vi "single_pulse_config.vi"(1 "output cluster":T1) -> (0 "Error output":T2)   [LabVIEW 2015]
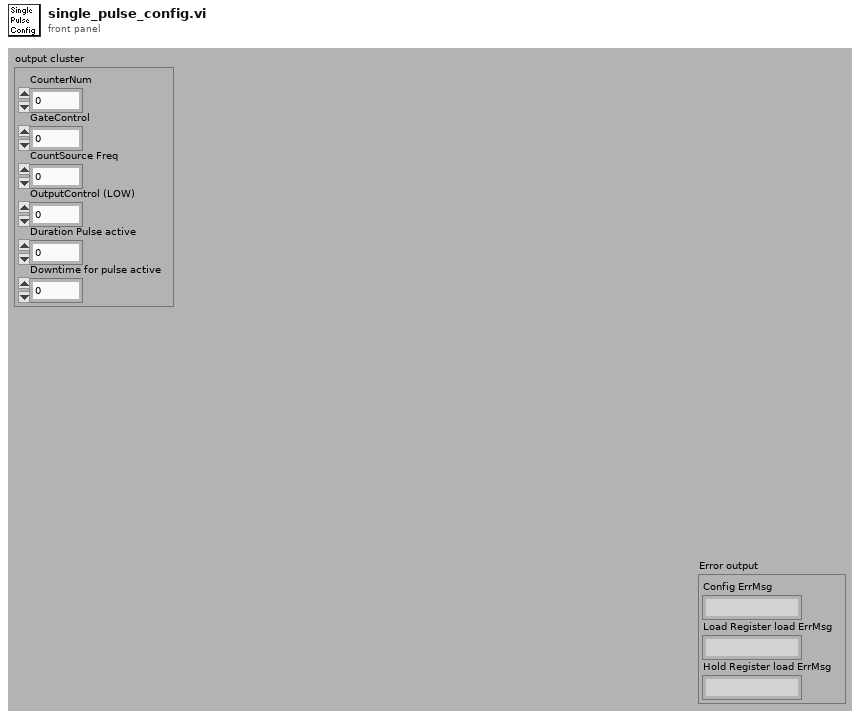
[diagram p1: front panel]
types:
  T1 = cluster{"CounterNum":u32, "GateControl":u32, "CountSource Freq":u32, "OutputControl (LOW)":u32, "Duration Pulse active":u32, "Downtime for pulse active":u32}
  T2 = cluster{"Config ErrMsg":string, "Load Register load ErrMsg":string, "Hold Register load ErrMsg":string}
  T3 = cluster{"ErrMsg":string, "ErrMsg":string, "ErrMsg":string}
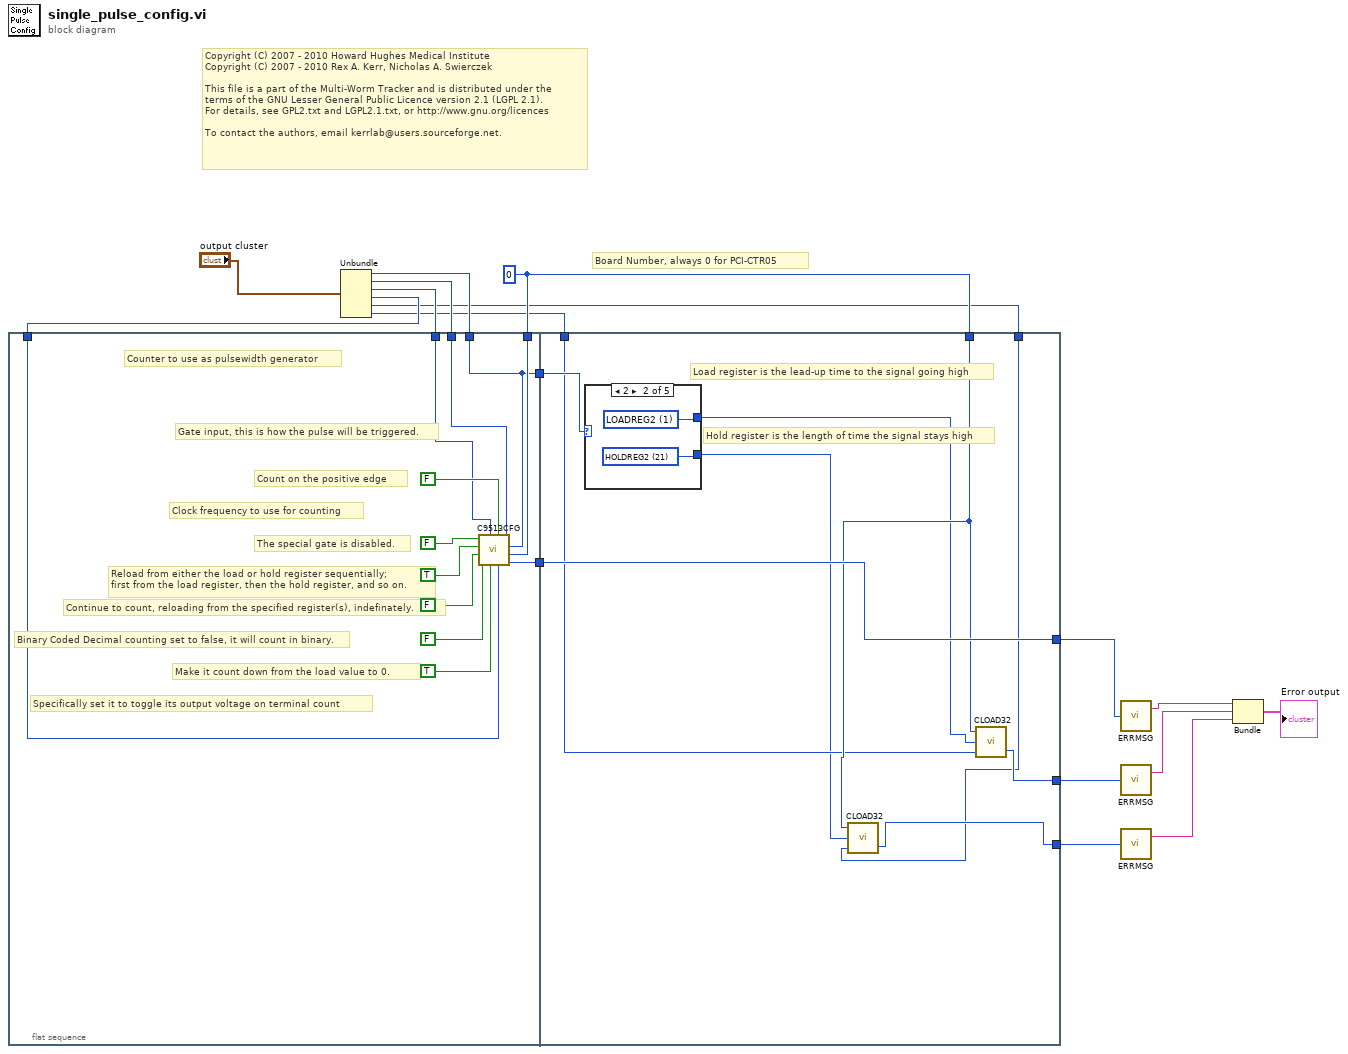
[diagram p0: block diagram]
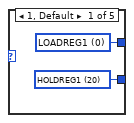
[diagram p2: hidden frame]
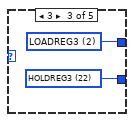
[diagram p3: hidden frame]
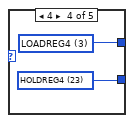
[diagram p4: hidden frame]
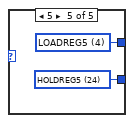
[diagram p5: hidden frame]
diagram:
  w9 = u32 0 ("BoardNum (0)")
  # "Copyright (C) 2007 - 2010 Howard Hughes Medical Institute\nCopyright (C) 2007 - 2010 Rex A. Kerr, Nicholas A. Swierczek\n \nThis file is a part of the Multi-Worm Tracker and is distributed under the\nterms of the GNU Lesser General Public Licence version 2.1 (LGPL 2.1).\nFor details, see GPL2.txt and LGPL2.1.txt, or http://www.gnu.org/licences\n \nTo contact the authors, email kerrlab@users.sourceforge.net."
  # "Board Number, always 0 for PCI-CTR05"
  n1 = flat-sequence {
    tunnel: [w23] -> w10
    tunnel: w9 -> [w22]
    tunnel: [w21] -> w8
    tunnel: w7 -> [w21]
    tunnel: w6 -> [w20]
    tunnel: w5 -> [w19]
    tunnel: w4 -> [w18]
    tunnel: [w38] -> w13
    tunnel: [w37] -> w12
    tunnel: [w36] -> w11
    tunnel: w10 -> [w36]
    tunnel: w9 -> [w35]
    tunnel: w8 -> [w33]
    tunnel: w3 -> [w32]
    tunnel: w2 -> [w31]
    frame #0 {
      # "Continue to count, reloading from the specified register(s), indefinately."
      # "Specifically set it to toggle its output voltage on terminal count"
      # "Make it count down from the load value to 0."
      # "Binary Coded Decimal counting set to false, it will count in binary."
      # "Reload from either the load or hold register sequentially;\nfirst from the load register, then the hold register, and so on."
      # "The special gate is disabled."
      # "Clock frequency to use for counting"
      # "Count on the positive edge"
      # "Gate input, this is how the pulse will be triggered."
      # "Counter to use as pulsewidth generator"
      n2 = call <menus>:"C9513CFG.VI"("BCDMode (DISABLED)"=FALSE, "CountDirection (UP)"=TRUE, "OutputControl (LOW)"=w18, "Recycle (ONETIME)"=FALSE, "BoardNum (0)"=w22, "Reload (LOADREG)"=TRUE, "CounterNum (1)"=w21, "SpecialGate (DISABLED)"=FALSE, "CountSource"=w19, "CountEdge(POSITIVE)"=FALSE, "GateControl"=w20) -> ("ErrCode"=w23:i32)
    }
    frame #1 {
      # "Load register is the lead-up time to the signal going high"
      # "Hold register is the length of time the signal stays high"
      n3 = case shown="2" w33 {
        tunnel: [w40 w42 w44 w46 w48] -> w34
        tunnel: [w39 w41 w43 w45 w47] -> w30
        frame 1, Default {
          w39 = u32 20 items=["LOADREG1", "LOADREG2", "LOADREG3", "LOADREG4", "LOADREG5", "LOADREG6", "LOADREG7", "LOADREG8", "LOADREG9", "LOADREG10", "LOADREG11", "LOADREG12", "LOADREG13", "LOADREG14", "LOADREG15", "LOADREG16", "LOADREG17", "LOADREG18", "LOADREG19", "LOADREG20", "HOLDREG1", "HOLDREG2", "HOLDREG3", "HOLDREG4", "HOLDREG5", "HOLDREG6", "HOLDREG7", "HOLDREG8", "HOLDREG9", "HOLDREG10", "HOLDREG11", "HOLDREG12", "HOLDREG13", "HOLDREG14", "HOLDREG15", "HOLDREG16", "HOLDREG17", "HOLDREG18", "HOLDREG19", "HOLDREG20", "ALARM1CHIP1", "ALARM2CHIP1", "ALARM1CHIP2", "ALARM2CHIP2", "ALARM1CHIP3", "ALARM2CHIP3", "ALARM1CHIP4", "ALARM2CHIP4", "COUNT1", "COUNT2", "COUNT3", "COUNT4", "PRESET1", "PRESET2", "PRESET3", "PRESET4", "PRESCALER1", "PRESCALER2", "PRESCALER3", "PRESCALER4"] ("Counter 1 Hold RegName")
          w40 = u32 0 items=["LOADREG1", "LOADREG2", "LOADREG3", "LOADREG4", "LOADREG5", "LOADREG6", "LOADREG7", "LOADREG8", "LOADREG9", "LOADREG10", "LOADREG11", "LOADREG12", "LOADREG13", "LOADREG14", "LOADREG15", "LOADREG16", "LOADREG17", "LOADREG18", "LOADREG19", "LOADREG20", "HOLDREG1", "HOLDREG2", "HOLDREG3", "HOLDREG4", "HOLDREG5", "HOLDREG6", "HOLDREG7", "HOLDREG8", "HOLDREG9", "HOLDREG10", "HOLDREG11", "HOLDREG12", "HOLDREG13", "HOLDREG14", "HOLDREG15", "HOLDREG16", "HOLDREG17", "HOLDREG18", "HOLDREG19", "HOLDREG20", "ALARM1CHIP1", "ALARM2CHIP1", "ALARM1CHIP2", "ALARM2CHIP2", "ALARM1CHIP3", "ALARM2CHIP3", "ALARM1CHIP4", "ALARM2CHIP4", "COUNT1", "COUNT2", "COUNT3", "COUNT4", "PRESET1", "PRESET2", "PRESET3", "PRESET4", "PRESCALER1", "PRESCALER2", "PRESCALER3", "PRESCALER4"] ("Counter 1 Load RegName")
        }
        frame 2 {
          w41 = u32 21 items=["LOADREG1", "LOADREG2", "LOADREG3", "LOADREG4", "LOADREG5", "LOADREG6", "LOADREG7", "LOADREG8", "LOADREG9", "LOADREG10", "LOADREG11", "LOADREG12", "LOADREG13", "LOADREG14", "LOADREG15", "LOADREG16", "LOADREG17", "LOADREG18", "LOADREG19", "LOADREG20", "HOLDREG1", "HOLDREG2", "HOLDREG3", "HOLDREG4", "HOLDREG5", "HOLDREG6", "HOLDREG7", "HOLDREG8", "HOLDREG9", "HOLDREG10", "HOLDREG11", "HOLDREG12", "HOLDREG13", "HOLDREG14", "HOLDREG15", "HOLDREG16", "HOLDREG17", "HOLDREG18", "HOLDREG19", "HOLDREG20", "ALARM1CHIP1", "ALARM2CHIP1", "ALARM1CHIP2", "ALARM2CHIP2", "ALARM1CHIP3", "ALARM2CHIP3", "ALARM1CHIP4", "ALARM2CHIP4", "COUNT1", "COUNT2", "COUNT3", "COUNT4", "PRESET1", "PRESET2", "PRESET3", "PRESET4", "PRESCALER1", "PRESCALER2", "PRESCALER3", "PRESCALER4"] ("Counter 1 Hold RegName")
          w42 = u32 1 items=["LOADREG1", "LOADREG2", "LOADREG3", "LOADREG4", "LOADREG5", "LOADREG6", "LOADREG7", "LOADREG8", "LOADREG9", "LOADREG10", "LOADREG11", "LOADREG12", "LOADREG13", "LOADREG14", "LOADREG15", "LOADREG16", "LOADREG17", "LOADREG18", "LOADREG19", "LOADREG20", "HOLDREG1", "HOLDREG2", "HOLDREG3", "HOLDREG4", "HOLDREG5", "HOLDREG6", "HOLDREG7", "HOLDREG8", "HOLDREG9", "HOLDREG10", "HOLDREG11", "HOLDREG12", "HOLDREG13", "HOLDREG14", "HOLDREG15", "HOLDREG16", "HOLDREG17", "HOLDREG18", "HOLDREG19", "HOLDREG20", "ALARM1CHIP1", "ALARM2CHIP1", "ALARM1CHIP2", "ALARM2CHIP2", "ALARM1CHIP3", "ALARM2CHIP3", "ALARM1CHIP4", "ALARM2CHIP4", "COUNT1", "COUNT2", "COUNT3", "COUNT4", "PRESET1", "PRESET2", "PRESET3", "PRESET4", "PRESCALER1", "PRESCALER2", "PRESCALER3", "PRESCALER4"] ("Counter 1 Load RegName")
        }
        frame 3 {
          w43 = u32 22 items=["LOADREG1", "LOADREG2", "LOADREG3", "LOADREG4", "LOADREG5", "LOADREG6", "LOADREG7", "LOADREG8", "LOADREG9", "LOADREG10", "LOADREG11", "LOADREG12", "LOADREG13", "LOADREG14", "LOADREG15", "LOADREG16", "LOADREG17", "LOADREG18", "LOADREG19", "LOADREG20", "HOLDREG1", "HOLDREG2", "HOLDREG3", "HOLDREG4", "HOLDREG5", "HOLDREG6", "HOLDREG7", "HOLDREG8", "HOLDREG9", "HOLDREG10", "HOLDREG11", "HOLDREG12", "HOLDREG13", "HOLDREG14", "HOLDREG15", "HOLDREG16", "HOLDREG17", "HOLDREG18", "HOLDREG19", "HOLDREG20", "ALARM1CHIP1", "ALARM2CHIP1", "ALARM1CHIP2", "ALARM2CHIP2", "ALARM1CHIP3", "ALARM2CHIP3", "ALARM1CHIP4", "ALARM2CHIP4", "COUNT1", "COUNT2", "COUNT3", "COUNT4", "PRESET1", "PRESET2", "PRESET3", "PRESET4", "PRESCALER1", "PRESCALER2", "PRESCALER3", "PRESCALER4"] ("Counter 1 Hold RegName")
          w44 = u32 2 items=["LOADREG1", "LOADREG2", "LOADREG3", "LOADREG4", "LOADREG5", "LOADREG6", "LOADREG7", "LOADREG8", "LOADREG9", "LOADREG10", "LOADREG11", "LOADREG12", "LOADREG13", "LOADREG14", "LOADREG15", "LOADREG16", "LOADREG17", "LOADREG18", "LOADREG19", "LOADREG20", "HOLDREG1", "HOLDREG2", "HOLDREG3", "HOLDREG4", "HOLDREG5", "HOLDREG6", "HOLDREG7", "HOLDREG8", "HOLDREG9", "HOLDREG10", "HOLDREG11", "HOLDREG12", "HOLDREG13", "HOLDREG14", "HOLDREG15", "HOLDREG16", "HOLDREG17", "HOLDREG18", "HOLDREG19", "HOLDREG20", "ALARM1CHIP1", "ALARM2CHIP1", "ALARM1CHIP2", "ALARM2CHIP2", "ALARM1CHIP3", "ALARM2CHIP3", "ALARM1CHIP4", "ALARM2CHIP4", "COUNT1", "COUNT2", "COUNT3", "COUNT4", "PRESET1", "PRESET2", "PRESET3", "PRESET4", "PRESCALER1", "PRESCALER2", "PRESCALER3", "PRESCALER4"] ("Counter 1 Load RegName")
        }
        frame 4 {
          w45 = u32 23 items=["LOADREG1", "LOADREG2", "LOADREG3", "LOADREG4", "LOADREG5", "LOADREG6", "LOADREG7", "LOADREG8", "LOADREG9", "LOADREG10", "LOADREG11", "LOADREG12", "LOADREG13", "LOADREG14", "LOADREG15", "LOADREG16", "LOADREG17", "LOADREG18", "LOADREG19", "LOADREG20", "HOLDREG1", "HOLDREG2", "HOLDREG3", "HOLDREG4", "HOLDREG5", "HOLDREG6", "HOLDREG7", "HOLDREG8", "HOLDREG9", "HOLDREG10", "HOLDREG11", "HOLDREG12", "HOLDREG13", "HOLDREG14", "HOLDREG15", "HOLDREG16", "HOLDREG17", "HOLDREG18", "HOLDREG19", "HOLDREG20", "ALARM1CHIP1", "ALARM2CHIP1", "ALARM1CHIP2", "ALARM2CHIP2", "ALARM1CHIP3", "ALARM2CHIP3", "ALARM1CHIP4", "ALARM2CHIP4", "COUNT1", "COUNT2", "COUNT3", "COUNT4", "PRESET1", "PRESET2", "PRESET3", "PRESET4", "PRESCALER1", "PRESCALER2", "PRESCALER3", "PRESCALER4"] ("Counter 1 Hold RegName")
          w46 = u32 3 items=["LOADREG1", "LOADREG2", "LOADREG3", "LOADREG4", "LOADREG5", "LOADREG6", "LOADREG7", "LOADREG8", "LOADREG9", "LOADREG10", "LOADREG11", "LOADREG12", "LOADREG13", "LOADREG14", "LOADREG15", "LOADREG16", "LOADREG17", "LOADREG18", "LOADREG19", "LOADREG20", "HOLDREG1", "HOLDREG2", "HOLDREG3", "HOLDREG4", "HOLDREG5", "HOLDREG6", "HOLDREG7", "HOLDREG8", "HOLDREG9", "HOLDREG10", "HOLDREG11", "HOLDREG12", "HOLDREG13", "HOLDREG14", "HOLDREG15", "HOLDREG16", "HOLDREG17", "HOLDREG18", "HOLDREG19", "HOLDREG20", "ALARM1CHIP1", "ALARM2CHIP1", "ALARM1CHIP2", "ALARM2CHIP2", "ALARM1CHIP3", "ALARM2CHIP3", "ALARM1CHIP4", "ALARM2CHIP4", "COUNT1", "COUNT2", "COUNT3", "COUNT4", "PRESET1", "PRESET2", "PRESET3", "PRESET4", "PRESCALER1", "PRESCALER2", "PRESCALER3", "PRESCALER4"] ("Counter 1 Load RegName")
        }
        frame 5 {
          w47 = u32 24 items=["LOADREG1", "LOADREG2", "LOADREG3", "LOADREG4", "LOADREG5", "LOADREG6", "LOADREG7", "LOADREG8", "LOADREG9", "LOADREG10", "LOADREG11", "LOADREG12", "LOADREG13", "LOADREG14", "LOADREG15", "LOADREG16", "LOADREG17", "LOADREG18", "LOADREG19", "LOADREG20", "HOLDREG1", "HOLDREG2", "HOLDREG3", "HOLDREG4", "HOLDREG5", "HOLDREG6", "HOLDREG7", "HOLDREG8", "HOLDREG9", "HOLDREG10", "HOLDREG11", "HOLDREG12", "HOLDREG13", "HOLDREG14", "HOLDREG15", "HOLDREG16", "HOLDREG17", "HOLDREG18", "HOLDREG19", "HOLDREG20", "ALARM1CHIP1", "ALARM2CHIP1", "ALARM1CHIP2", "ALARM2CHIP2", "ALARM1CHIP3", "ALARM2CHIP3", "ALARM1CHIP4", "ALARM2CHIP4", "COUNT1", "COUNT2", "COUNT3", "COUNT4", "PRESET1", "PRESET2", "PRESET3", "PRESET4", "PRESCALER1", "PRESCALER2", "PRESCALER3", "PRESCALER4"] ("Counter 1 Hold RegName")
          w48 = u32 4 items=["LOADREG1", "LOADREG2", "LOADREG3", "LOADREG4", "LOADREG5", "LOADREG6", "LOADREG7", "LOADREG8", "LOADREG9", "LOADREG10", "LOADREG11", "LOADREG12", "LOADREG13", "LOADREG14", "LOADREG15", "LOADREG16", "LOADREG17", "LOADREG18", "LOADREG19", "LOADREG20", "HOLDREG1", "HOLDREG2", "HOLDREG3", "HOLDREG4", "HOLDREG5", "HOLDREG6", "HOLDREG7", "HOLDREG8", "HOLDREG9", "HOLDREG10", "HOLDREG11", "HOLDREG12", "HOLDREG13", "HOLDREG14", "HOLDREG15", "HOLDREG16", "HOLDREG17", "HOLDREG18", "HOLDREG19", "HOLDREG20", "ALARM1CHIP1", "ALARM2CHIP1", "ALARM1CHIP2", "ALARM2CHIP2", "ALARM1CHIP3", "ALARM2CHIP3", "ALARM1CHIP4", "ALARM2CHIP4", "COUNT1", "COUNT2", "COUNT3", "COUNT4", "PRESET1", "PRESET2", "PRESET3", "PRESET4", "PRESCALER1", "PRESCALER2", "PRESCALER3", "PRESCALER4"] ("Counter 1 Load RegName")
        }
      }
      n4 = call <menus>:"CLOAD32.VI"("LoadValue"=w32, "RegName"=w30, "BoardNum (0)"=w35) -> ("ErrCode"=w37:i32)  [unwired: 1 out]
      n5 = call <menus>:"CLOAD32.VI"("LoadValue"=w31, "RegName"=w34, "BoardNum (0)"=w35) -> ("ErrCode"=w38:i32)  [unwired: 1 out]
    }
  }
  n6 = Unbundle("output cluster") -> ("CounterNum"=w7:u32, "GateControl"=w6:u32, "CountSource Freq"=w5:u32, "OutputControl (LOW)"=w4:u32, "Duration Pulse active"=w3:u32, "Downtime for pulse active"=w2:u32)
  n7 = call <menus>:"ERRMSG.VI"("ErrCode"=w11) -> ("ErrMsg"=w17:string)  [unwired: 1 out]
  n8 = call <menus>:"ERRMSG.VI"("ErrCode"=w13) -> ("ErrMsg"=w16:string)  [unwired: 1 out]
  n9 = call <menus>:"ERRMSG.VI"("ErrCode"=w12) -> ("ErrMsg"=w15:string)  [unwired: 1 out]
  n10 = Bundle("ErrMsg"=w17, "ErrMsg"=w16, "ErrMsg"=w15) -> (→"Error output":T3)  [unwired: 1 in]
